vi "Getting Started with OAT (Offline, Digital Tacho) .vi"() -> ()   [LabVIEW 2017]
doc: "<B>DESCRIPTIONS</B>:\nThis VI demonstrates how to perform basic order analysis functions such as speed calculation, vibration level measurement, spectral map, order power spectrum, and order magnitude and phase. It loads the recorded signals acquired with Log Data (Digital Tacho , DAQmx).vi for offline analysis. \n\n<B>INSTRUCTIONS</B>:\n1. Select the data file to load first.\n2. Run the VI.\n3. On the <B>Time Waveform and Speed Profile</B> tab, select the signal of interest in <B>select channel</B> and specify the <B>Start</B> and <B>Duration</B> of the signal to calculate sound or vibration level. Run th VI again to make the changes take effect.\n4. On the <B>Colormap</B> tab, select the signal of interest in <B>select channel</B>. Use the <B>plot type</B> control to change the type of colormap. Specify the <B>time segment</B> and <B>spectra settings</B> to get a better view of the colormap. Run the VI again to make the changes take effect.\n5. On the <B>Order Power Spectrum</B> tab, specify the <B>Start</B> and <B>Duration</B> of the signal to calculate the order power spectrum. Specify the <B>window type</B>, <B>block size</B> and <B>averaging parameters</B> to improve the order power spectrum calculation and display. Run the VI again to make the changes take effect.\n<B>Note</B>: when the <B>Duration</B> of the signal is too short, there may not be an order power spectrum output. In this case, you should increase the duration or decrease the <B>block size</B> to get the order power spectrum results.\n6. On the <B>Magnitude and Phase</B> tab, select the signal of interest in <B>select channel</B> and specify the order to calculate magnitude and phase in <B>orders to compute</B>. Change the <B>magnitude view</B> and <B>view</B> to gain desired magnitude and phase display formats. Run the VI again to make the changes take effect.\n\n<B>ORDER ANALYSIS VIs USED IN THIS EXAMPLE</B>:\n1. SVL Scale Voltage to EU.vi\n2. OAT Digital Tacho Process.vi\n3. SVL RMS Level.vi\n4. SVL Peak Level.vi\n5. OAT Spectral Map.vi\n6. OAT Convert to Even Angle Signal.vi\n7. OAT Order Power Spectrum.vi\n8. OAT Order Magnitude and Phase.vi\n9. SVL Unit Conversion.vi"
uses:
  <vilib>/addons/_XControls/Colormap/SVX Colormap.xctl
  <vilib>/addons/Sound and Vibration/svt_Calibration/SVL Scale Voltage to EU (1 Ch).vi
  <vilib>/addons/_NISVFA/_Shared subVIs/Common/svc_Set SV Channel Info.vi
  <vilib>/addons/_NISVFA/_Shared subVIs/Common/svc_Set SV Channel Info (variant).vi
  <vilib>/addons/_NISVFA/_Shared subVIs/Common/SVL Set dB Reference (variant).vi
  <vilib>/addons/_NISVFA/_Shared subVIs/Common/svc_Caller VI Returned in Error Source.vi
  <vilib>/addons/_NISVFA/_Shared subVIs/Common/svc_Engineering Units to Unit Label.vi
  <vilib>/addons/_NISVFA/_Shared subVIs/Common/svc_Set dB ref if Pascal.vi
  <vilib>/addons/_NISVFA/_Shared subVIs/Common/svc_Compute Scale Factor to Convert C to EU.vi
  <vilib>/addons/_NISVFA/_Shared subVIs/Common/svc_Compute Scale Factor to Convert V to EU.vi
  <vilib>/addons/Sound and Vibration/Order Analysis/Tach Process/SoundVib_TachProcess.lvlib
  <vilib>/addons/Sound and Vibration/svt_Calibration/SoundVib_Calibration.lvlib
  <vilib>/addons/Sound and Vibration/Order Analysis/Resample Order Tracking/SoundVib_OrderTracking.lvlib
panel:
  in  "Data Path":path
  out "fs":dbl=44100.0
  out "number of samples":i32=44100
  in  "Tab Control":T1(tab)
  out "Peak level [EU]":dbl format="%.2f"
  in  "Duration":dbl=1.0 format="%0.2f"
  in  "Start":dbl format="%0.2f"
  in  "select channel":u16(ring) items=["PC fan runup"]
  out "RMS level [EU]":dbl format="%.2f"
  in  "max order to analyze":dbl=32.0
  out "Speed profile":cluster{"time [s]":dbl[], "speed [RPM]":dbl[]}(graph)
  out "Vibration signals":waveform(dbl)(graph)
  in  "plot type":T2(ring)
  in  "time segment":T3={"start [s]"=0.0, "end [s]"=inf, "step size [s]"=0.05} {"step size [s]" format="%.2f"; "end [s]" format="%.2f"; "start [s]" format="%.2f"}
  in  "select channel":u16(ring) items=["PC fan runup"]
  in  "spectra settings":T4={"window type"=62, "freq/order bins"=2048} {"freq/order bins" min=2; "window type" items=["None"=0, "Hanning"=1, "Hamming"=2, "Blackman-Harris"=3, "Exact Blackman"=4, "Blackman"=5, "Flat Top"=6, "4 Term B-Harris"=7, "7 Term B-Harris"=8, "Low Sidelobe"=9, "Gaussian"=62]}
  in  "dB On":bool=TRUE
  out "colormap":T5(xcontrol) caption="Colormap"
  in  "Duration":dbl=10.0 format="%0.2f"
  in  "Start":dbl format="%0.2f"
  in  "averaging parameters":T6={"averaging mode"=enum."RMS averaging", "weighting mode"=enum."Exponential", "number of averages"=10, "linear mode"=enum."One shot"} {"number of averages" min=1 step=1}
  in  "block size":i32=1024 min=2
  in  "window type":u32(ring)=1 items=["None"=0, "Hanning"=1, "Hamming"=2, "Blackman-Harris"=3, "Exact Blackman"=4, "Blackman"=5, "Flat Top"=6, "4 Term B-Harris"=7, "7 Term B-Harris"=8, "Low Sidelobe"=9, "Gaussian"=62]
  in  "dB On":bool=TRUE
  out "Order Power Spectrum":T7(graph) caption="Order power spectrum"
  in  "view":T8={"dB on? (F)"=FALSE, "unwrap phase? (T)"=TRUE, "unit in degree? (T)"=TRUE}
  in  "magnitude view":enum16{"no change", "rms", "peak", "peak-peak"}(ring)
  in  "select channel":u16(ring) items=["PC fan runup"]
  in  "X axis selection":u16(ring) items=["Time", "Revolution", "RPM"]
  in  "bandwidth [order]":dbl format="%.2f"
  in  "orders to compute":dbl[](array[numeric])=[1.0] format="%.2f"
  out "Phase":cluster{"time/rev/rpm":dbl[], "phase":dbl[]}[](graph)
  out "Magnitude":T9(graph)
  # "Select Help»Show Context Help and move the cursor over the VI icon for more information."
  # "Vibration Level Measurement"
  # "select data block"
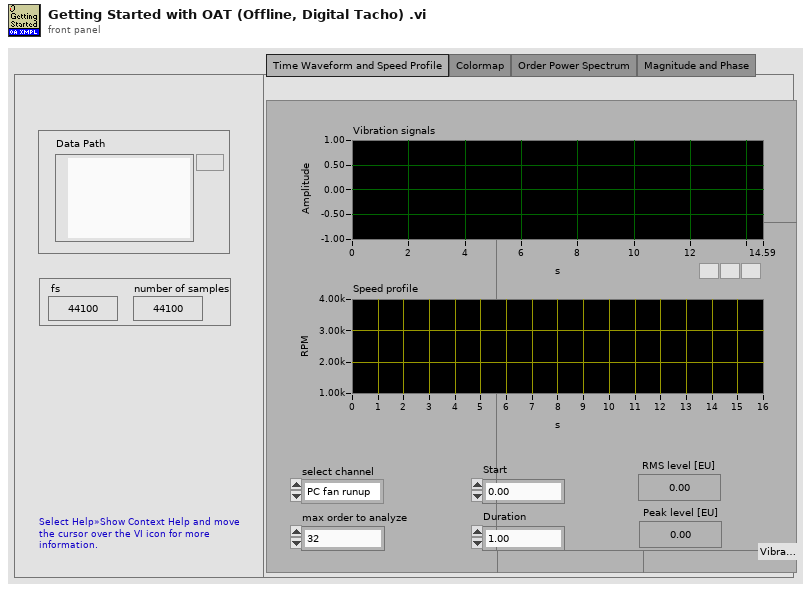
[diagram p1: front panel]
types:
  T1 = enum32{"Time Waveform and Speed Profile", "Colormap", "Order Power Spectrum", "Magnitude and Phase"}
  T2 = enum16{"Frequency-Time", "Time-Frequency", "Order-Time", "Time-Order", "Frequency-RPM", "RPM-Frequency", "Order-RPM", "RPM-Order"}
  T3 = cluster{"start [s]":dbl, "end [s]":dbl, "step size [s]":dbl}
  T4 = cluster{"window type":u32, "freq/order bins":i32}
  T5 = cluster{"spectral map":dbl[][], "X scale":cluster{"offset":dbl, "multiplier":dbl}, "Y scale":cluster{"offset":dbl, "multiplier":dbl}, "attribute":variant}
  T6 = cluster{"averaging mode":enum16{"No averaging", "Vector averaging", "RMS averaging", "Peak hold"}, "weighting mode":enum16{"Linear", "Exponential"}, "number of averages":u32, "linear mode":enum16{"One shot", "Auto restart"}}
  T7 = cluster{"order 0":dbl, "delta order":dbl, "magnitude":dbl[]}[]
  T8 = cluster{"dB on? (F)":bool, "unwrap phase? (T)":bool, "unit in degree? (T)":bool}
  T9 = cluster{"time/rev/rpm":dbl[], "magnitude":dbl[]}[]
  T10 = typedef "svc_Channel Info.ctl" = cluster{"sensor sensitivity":dbl, "engineering units":T11, "dB reference":dbl, "custom label":string, "weighting filter":T12, "pregain":dbl}
  T11 = typedef "svc_Engineering Units Text Ring.ctl" = u16
  T12 = typedef "svc_Weighting Filter Text Ring.ctl" = u16
  T13 = typedef "SoundVib_TachProcess.lvlib/digital tach info.ctl" = cluster{"tacho counts":i64[], "counter timebase [Hz]":dbl, "counter task type":enum16{"period measurement", "event counting"}, "counter digit (32)":i32}
  T14 = typedef "SoundVib_TachProcess.lvlib/speed profile.ctl" = cluster{"time [s]":dbl[], "speed [RPM]":dbl[]}
  T15 = cluster{"value":dbl[][], "x scale":cluster{"offset":dbl, "multiplier":dbl}, "y scale":cluster{"offset":dbl, "multiplier":dbl}, "attribute":variant}
  T16 = cluster{"x-axis unit label":string, "y-axis unit label":string, "z-axis unit label":string}
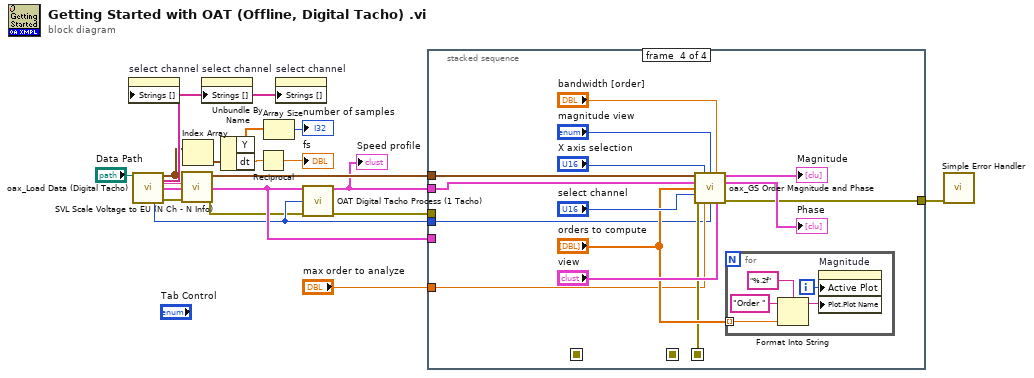
[diagram p0: block diagram]
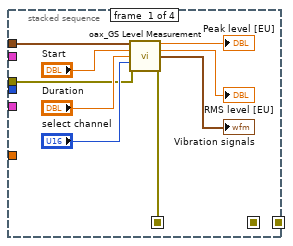
[diagram p2: hidden frame]
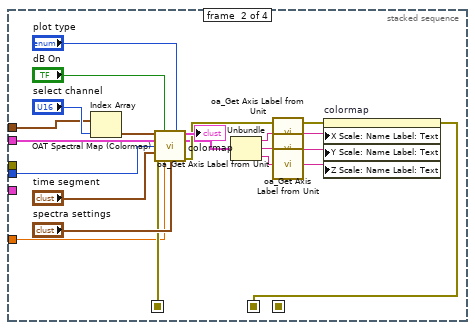
[diagram p3: hidden frame]
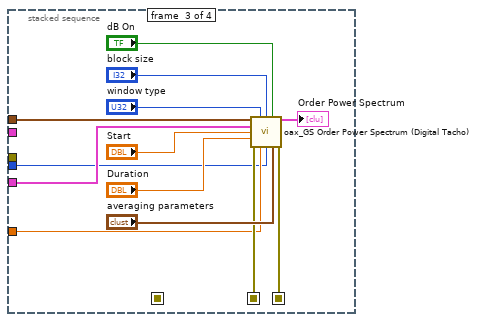
[diagram p4: hidden frame]
diagram:
  n1 = call <vilib>:"oax_Load Data (Digital Tacho).vi"("Data Path In"="Data Path") -> ("channel name"=w18:string[], "vibration data"=w11:waveform(dbl)[], "vibration channel info"=w9:T10[], "digital tacho info"=w6:T13, "pulse / rev"=w3:i32, "error out"=w12:errorcluster)  [unwired: 9 in]
  n2 = property on="select channel" class="Ring (strict)"("Strings []"=w18) -> ()  [unwired: 2 in, 2 out]
  n3 = call <vilib>:"SVL Scale Voltage to EU (N Ch - N Info).vi"("error in (no error)"=w12, "channel info"=w9, "signals [V]"=w11) -> ("error out"=w1:errorcluster, "scaled signals [EU]"=w8:waveform(dbl)[])  [unwired: 6 in, 1 out]
  n4 = Index Array(array=w11) -> (element=w10:waveform(dbl))  [unwired: 1 in]
  n5 = property on="select channel" class="Ring (strict)"("Strings []"=w18) -> ()  [unwired: 2 in, 2 out]
  n6 = Unbundle By Name(w10) -> ("Y"=w14:dbl[], "dt"=w16:dbl)
  n7 = Reciprocal(x=w16) -> (1/x=→"fs":dbl)
  n8 = Array Size(array=w14) -> (size(s)=→"number of samples":i32)
  n9 = property on="select channel" class="Ring (strict)"("Strings []"=w18) -> ()  [unwired: 2 in, 2 out]
  n10 = call <vilib>:"OAT Digital Tacho Process (1 Tacho).vi"("digital tacho info"=w6, "pulse/revolution (1)"=w3, "error in (no error)"=w1) -> ("speed profile"=w5:T14, "error out"=w7:errorcluster)  [unwired: 9 in, 2 out]
  "Speed profile" <- w5
  n11 = stacked-sequence {
    seq-local: [_ w36 _ _] -> [_ _ w52 _]
    seq-local: [_ _ w51 _] -> [_ _ _ w65]
    seq-local: [w19 _ _ _] -> [_ w43 _ _]
    tunnel: w8 -> [w21 w39 w54 w67]
    tunnel: w7 -> [w20 _ _ _]
    tunnel: w6 -> [_ _ w53 _]
    tunnel: w5 -> [_ w41 _ w66]
    tunnel: "max order to analyze" -> [_ w42 w50 w64]
    tunnel: w3 -> [_ w40 w49 w62]
    tunnel: [_ _ _ w63] -> w2
    frame #0 {
      n12 = call <vilib>:"oax_GS Level Measurement.vi"("scaled signals [EU]"=w21, "Start"="Start", "Duration"="Duration", "select channel"="select channel", "error in (no error)"=w20) -> ("Peak level [EU]"=→"Peak level [EU]":dbl, "RMS level [EU]"=→"RMS level [EU]":dbl, "vibration signals"=→"Vibration signals":waveform(dbl), "error out"=w19:errorcluster)  [unwired: 7 in]
    }
    frame #1 {
      n13 = Index Array(array=w39, index="select channel") -> (element=w45:waveform(dbl))
      n14 = call <vilib>:"OAT Spectral Map (Colormap).vi"("scaled signal [EU]"=w45, "dB on? (T)"="dB On", "plot type"="plot type", "speed profile"=w41, "pulse/revolution (1)"=w40, "time/speed segment [s or RPM]"="time segment", "error in (no error)"=w43, "max order (auto)"=w42, "windows info"="spectra settings") -> ("colormap"=→"colormap":T15, "colormap unit labels"=w35:T16, "error out"=w37:errorcluster)  [unwired: 2 in, 2 out]
      n15 = Unbundle(w35) -> ("x-axis unit label"=w31:string, "y-axis unit label"=w33:string, "z-axis unit label"=w29:string)
      n16 = call <vilib>:"oa_Get Axis Label from Unit.vi"("Unit"=w31) -> ("Label"=w32:string)  [unwired: 4 in]
      n17 = call <vilib>:"oa_Get Axis Label from Unit.vi"("Unit"=w33) -> ("Label"=w30:string)  [unwired: 4 in]
      n18 = call <vilib>:"oa_Get Axis Label from Unit.vi"("Unit"=w29) -> ("Label"=w28:string)  [unwired: 4 in]
      n19 = property on="colormap" class="Colormap (strict)"(error in=w37, "X Scale: Name Label: Text"=w32, "Y Scale: Name Label: Text"=w30, "Z Scale: Name Label: Text"=w28) -> (error out=w36:errorcluster)  [unwired: 1 in, 1 out]
    }
    frame #2 {
      n20 = call <vilib>:"oax_GS Order Power Spectrum (Digital Tacho).vi"("scaled signals [EU]"=w54, "window type"="window type", "block size"="block size", "dB On"="dB On", "digital tacho info"=w53, "Start"="Start", "Duration"="Duration", "error in (no error)"=w52, "max order to analyze"=w50, "pulse/rev"=w49, "averaging parameters"="averaging parameters") -> ("Order Power Spectrum"=→"Order Power Spectrum":T7, "error out"=w51:errorcluster)  [unwired: 3 in]
    }
    frame #3 {
      n21 = call <vilib>:"oax_GS Order Magnitude and Phase.vi"("scaled signals [EU]"=w67, "X axis selection"="X axis selection", "magnitude view"="magnitude view", "bandwidth [order]"="bandwidth [order]", "speed profile"=w66, "orders to track"="orders to compute", "select channel"="select channel", "error in (no error)"=w65, "max order to analyze"=w64, "pulse/rev"=w62, "view"="view") -> ("magnitude"=→"Magnitude":T9, "phase"=→"Phase":cluster{"time/rev/rpm":dbl[], "phase":dbl[]}[], "error out"=w63:errorcluster)  [unwired: 1 in, 1 out]
      n22 = for {
        tunnel: "orders to compute" -> [w80] mode=indexing
        i -> [w76]
        n23 = Format Into String(format string="%.2f" ("Format String"), initial string="Order " ("Input String"), w80) -> (resulting string=w77:string)  [unwired: 1 in, 1 out]
        n24 = property on="Magnitude" class="XYGraph (strict)"("Active Plot"=w76, "Plot.Plot Name"=w77) -> ()  [unwired: 2 in, 2 out]
      }
    }
  }
  n25 = call <vilib>:"Simple Error Handler.vi"("error in (no error)"=w2) -> ()  [unwired: 4 in, 5 out]
